vi "MultitaskExample.vi"() -> ()   [LabVIEW 2017]
uses:
  <vilib>/FPGAPlugInAG/sbRIO-9607/niLvFpga_Open_sbRIO-9607.vi
  <vilib>/rvi/interface/common/dynamic/niFpgaDynamicAddResources.vi
  <vilib>/FPGAPlugInAG/Dynamic/niLvFpga_Reset_Dynamic.vi
  <vilib>/FPGAPlugInAG/Dynamic/niLvFpga_Run_Dynamic.vi
  RT/ReadWaveform.vi
  RT/Read2D.vi
  <vilib>/Utility/error.llb/Error Cluster From Error Code.vi
  <vilib>/rvi/errors/niLvFpgaAdjustHostInterfaceError.vi
  <vilib>/FPGAPlugInAG/Dynamic/niLvFpga_Close_Dynamic.vi
  <vilib>/rvi/interface/nirviOpenFPGA/nirviOpenFPGA.xnode
  FPGA Bitfiles/WaveformLibraryI_FPGATarget2_[FPGA]SARAcqMain_U+qOsuK4w1s.lvbitx
  <vilib>/rvi/interface/nirviMethod/nirviMethod.xnode
  <vilib>/rvi/interface/nirviReadWriteControl/nirviReadWriteControl.xnode
  <vilib>/rvi/interface/nirviCloseFPGA/nirviCloseFPGA.xnode
  <instrlib>/_niInstr/FIFO Register Bus/v1/Host/niInstr FIFO Register Bus v1 Host.lvclass
  RT/WaveformTask.lvclass
  NiFpgaLv.dll
  <vilib>/rvi/interface/Simulation/niFpgaSimulationCallBeginRW.vi
panel:
  in  "stop":bool
  in  "injectError0":errorcluster
  out "Data 4":waveform(sgl)[](graph)
  out "Data 3":sgl[][](graph)
  out "Data 2":sgl[][](graph)
  out "Data":waveform(sgl)[](graph)
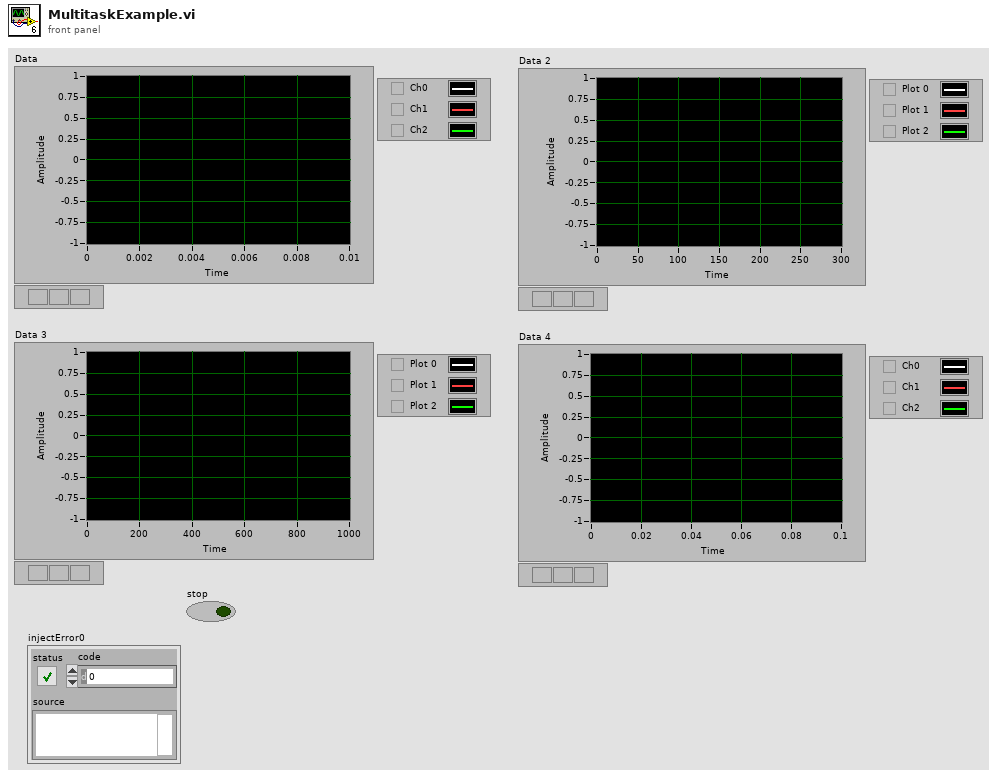
[diagram p1: front panel]
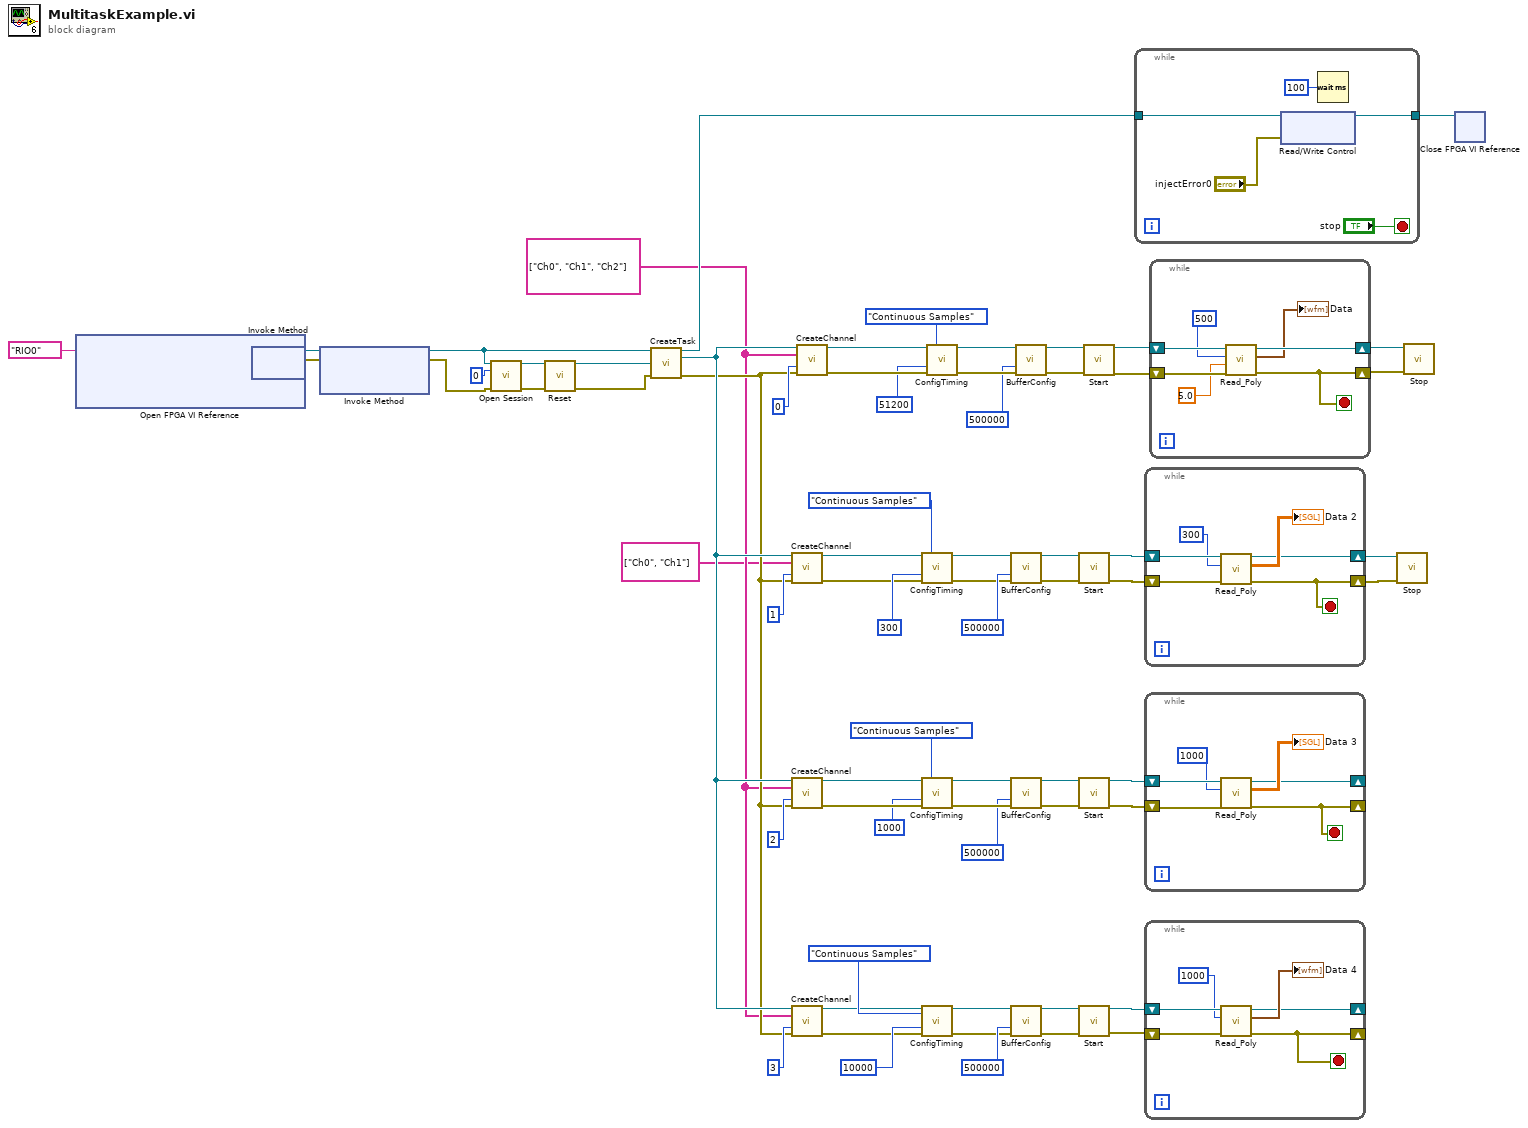
[diagram p0: block diagram]
diagram:
  w2 = string[] ["Ch0", "Ch1", "Ch2"] ("Chan Name Array")
  n1 = xnode "Open FPGA VI Reference"("resource name"=tag "RIO0") -> ("FPGA VI Reference Out"=w58:refnum<k20>, "error out"=w57:errorcluster)  [unwired: 1 in]
  n2 = xnode "Invoke Method"("FPGA VI Reference In"=w58, "error in"=w57) -> ("FPGA VI Reference Out"=w56:refnum<k20>, "error out"=w55:errorcluster)
  n3 = xnode "Invoke Method"("FPGA VI Reference In"=w56, "error in"=w55) -> ("FPGA VI Reference Out"=w5:refnum<k20>, "error out"=w6:errorcluster)  [unwired: 1 in]
  n4 = call <instrlib>:"Open Session.vi"("fpga ref"=w5, "bus instance"=u32 0, "error in"=w6) -> ("session out"=w8:refnum<class "niInstr FIFO Register Bus v1 Host.lvclass">, "error out"=w9:errorcluster)  [unwired: 11 in]
  n5 = call-dynamic "Reset.vi"("session in"=w8, "error in"=w9) -> ("session out"=w4:refnum<class "niInstr FIFO Register Bus v1 Host.lvclass">, "error out"=w3:errorcluster)  [unwired: 12 in]
  n6 = call "CreateTask.vi"("FPGA Ref in"=w5, "session in"=w4, "error in"=w3) -> ("FPGA Ref out"=w41:refnum<k20>, "Task out"=w16:refnum<class "WaveformTask.lvclass">, "error out"=w15:errorcluster)  [unwired: 9 in, 1 out]
  n7 = call "CreateChannel.vi"("task in"=w16, "Chan Name Array"=string[] ["Ch0", "Ch1"], "instance"=u8 1, "error in"=w15) -> ("Task out"=w42:refnum<class "WaveformTask.lvclass">, "error out"=w45:errorcluster)  [unwired: 10 in]
  n8 = call "CreateChannel.vi"("task in"=w16, "Chan Name Array"=w2, "instance"=u8 2, "error in"=w15) -> ("Task out"=w40:refnum<class "WaveformTask.lvclass">, "error out"=w38:errorcluster)  [unwired: 10 in]
  n9 = call "CreateChannel.vi"("task in"=w16, "Chan Name Array"=w2, "instance"=u8 3, "error in"=w15) -> ("Task out"=w17:refnum<class "WaveformTask.lvclass">, "error out"=w19:errorcluster)  [unwired: 10 in]
  n10 = call "CreateChannel.vi"("task in"=w16, "Chan Name Array"=w2, "instance"=u8 0, "error in"=w15) -> ("Task out"=w43:refnum<class "WaveformTask.lvclass">, "error out"=w68:errorcluster)  [unwired: 10 in]
  n11 = call "ConfigTiming.vi"("Task in"=w42, "Sample Mode"=enum16{"Finite Samples", "Continuous Samples"}."Continuous Samples", "Sample Rate"=u32 300, "error in (no error)"=w45) -> ("Task out"=w48:refnum<class "WaveformTask.lvclass">, "error out"=w49:errorcluster)  [unwired: 9 in, 1 out]
  n12 = call "ConfigTiming.vi"("Task in"=w40, "Sample Mode"=enum16{"Finite Samples", "Continuous Samples"}."Continuous Samples", "Sample Rate"=u32 1000, "error in (no error)"=w38) -> ("Task out"=w35:refnum<class "WaveformTask.lvclass">, "error out"=w34:errorcluster)  [unwired: 9 in, 1 out]
  n13 = call "ConfigTiming.vi"("Task in"=w17, "Sample Mode"=enum16{"Finite Samples", "Continuous Samples"}."Continuous Samples", "Sample Rate"=u32 10000, "error in (no error)"=w19) -> ("Task out"=w22:refnum<class "WaveformTask.lvclass">, "error out"=w23:errorcluster)  [unwired: 9 in, 1 out]
  n14 = call "ConfigTiming.vi"("Task in"=w43, "Sample Mode"=enum16{"Finite Samples", "Continuous Samples"}."Continuous Samples", "Sample Rate"=u32 51200, "error in (no error)"=w68) -> ("Task out"=w65:refnum<class "WaveformTask.lvclass">, "error out"=w64:errorcluster)  [unwired: 9 in, 1 out]
  n15 = call "BufferConfig.vi"("WaveformTask in"=w48, "Buffer Size [Samps per Chan]"=500000, "error in (no error)"=w49) -> ("WaveformTask out"=w51:refnum<class "WaveformTask.lvclass">, "error out"=w52:errorcluster)  [unwired: 10 in, 1 out]
  n16 = call "BufferConfig.vi"("WaveformTask in"=w35, "Buffer Size [Samps per Chan]"=500000, "error in (no error)"=w34) -> ("WaveformTask out"=w32:refnum<class "WaveformTask.lvclass">, "error out"=w31:errorcluster)  [unwired: 10 in, 1 out]
  n17 = call "BufferConfig.vi"("WaveformTask in"=w22, "Buffer Size [Samps per Chan]"=500000, "error in (no error)"=w23) -> ("WaveformTask out"=w25:refnum<class "WaveformTask.lvclass">, "error out"=w26:errorcluster)  [unwired: 10 in, 1 out]
  n18 = call "BufferConfig.vi"("WaveformTask in"=w65, "Buffer Size [Samps per Chan]"=500000, "error in (no error)"=w64) -> ("WaveformTask out"=w62:refnum<class "WaveformTask.lvclass">, "error out"=w61:errorcluster)  [unwired: 10 in, 1 out]
  n19 = call "Start.vi"("WaveformTask in"=w51, "error in (no error)"=w52) -> ("WaveformTask out"=w53:refnum<class "WaveformTask.lvclass">, "error out"=w54:errorcluster)  [unwired: 12 in]
  n20 = call "Start.vi"("WaveformTask in"=w32, "error in (no error)"=w31) -> ("WaveformTask out"=w30:refnum<class "WaveformTask.lvclass">, "error out"=w29:errorcluster)  [unwired: 12 in]
  n21 = call "Start.vi"("WaveformTask in"=w25, "error in (no error)"=w26) -> ("WaveformTask out"=w27:refnum<class "WaveformTask.lvclass">, "error out"=w28:errorcluster)  [unwired: 12 in]
  n22 = call "Start.vi"("WaveformTask in"=w62, "error in (no error)"=w61) -> ("WaveformTask out"=w60:refnum<class "WaveformTask.lvclass">, "error out"=w59:errorcluster)  [unwired: 12 in]
  n23 = while {
    tunnel: w41 -> [w73]
    tunnel: [w72] -> w10
    stop <- "stop" stop-if-true
    n24 = xnode "Read/Write Control"("FPGA VI Reference In"=w73, "injectError0"="injectError0") -> ("FPGA VI Reference Out"=w72:refnum<k20>)  [unwired: 1 in, 1 out]
    n25 = Wait (ms)(milliseconds to wait=u32 100) -> ()  [unwired: 1 out]
  }
  n26 = while {
    shift-right: [w76] -> w11
    shift-left: w54 -> [w80]
    shift-right: [w78] -> w12
    shift-left: w53 -> [w81]
    stop <- w76 stop-if-true
    n27 = call-poly "Read_Poly.vi"("error in"=w80, "Samps Read per Chan"=300, "Task in"=w81) -> ("error out"=w76:errorcluster, "Data"=→"Data 2":sgl[][], "Task out"=w78:refnum<class "WaveformTask.lvclass">)  [unwired: 5 in, 1 out]
  }
  n28 = while {
    shift-right: [w82] -> _
    shift-left: w29 -> [w86]
    shift-right: [w84] -> _
    shift-left: w30 -> [w87]
    stop <- w82 stop-if-true
    n29 = call-poly "Read_Poly.vi"("error in"=w86, "Samps Read per Chan"=1000, "Task in"=w87) -> ("error out"=w82:errorcluster, "Data"=→"Data 3":sgl[][], "Task out"=w84:refnum<class "WaveformTask.lvclass">)  [unwired: 5 in, 1 out]
  }
  n30 = while {
    shift-right: [w88] -> _
    shift-left: w28 -> [w92]
    shift-right: [w90] -> _
    shift-left: w27 -> [w93]
    stop <- w88 stop-if-true
    n31 = call-poly "Read_Poly.vi"("error in"=w92, "Samps Read per Chan"=1000, "Task in"=w93) -> ("error out"=w88:errorcluster, "Waveforms"=→"Data 4":waveform(sgl)[], "Task out"=w90:refnum<class "WaveformTask.lvclass">)  [unwired: 5 in, 1 out]
  }
  n32 = while {
    shift-right: [w94] -> w13
    shift-left: w59 -> [w99]
    shift-right: [w96] -> w14
    shift-left: w60 -> [w100]
    stop <- w94 stop-if-true
    n33 = call-poly "Read_Poly.vi"("error in"=w99, "Timeout (s)"=5.0, "Samps Read per Chan"=500, "Task in"=w100) -> ("error out"=w94:errorcluster, "Waveforms"=→"Data":waveform(sgl)[], "Task out"=w96:refnum<class "WaveformTask.lvclass">)  [unwired: 4 in, 1 out]
  }
  n34 = call "Stop.vi"("error in"=w11, "WaveformTask in"=w12) -> ()  [unwired: 8 in, 2 out]
  n35 = call "Stop.vi"("error in"=w13, "WaveformTask in"=w14) -> ()  [unwired: 8 in, 2 out]
  n36 = xnode "Close FPGA VI Reference"("FPGA VI Reference In"=w10) -> ()  [unwired: 1 in, 1 out]
